vi "test-DiffOdometry.vi"() -> ()   [LabVIEW 2019]
uses:
  POSE.ctl
  TRANSLATION.ctl
  ROTATION.ctl
  PATH_SAMPLE.ctl
  PathExecution_Library.lvlib
panel:
  in  "Ramsete Enable":bool=TRUE
  in  "WheelBase-Feet":dbl
  in  "Path Sample":T1
  out "RightDmd FT/SEC":dbl
  out "LeftDMD Ft?SEC":dbl
  out "Heading DEG":dbl
  out "AtReference":bool
  out "Y Feet":dbl
  out "X Feet":dbl
  out "CurrentRelativePose":T2
  in  "Reset":bool
  in  "Gyro-Deg":dbl
  in  "RightDist-Feet":dbl
  in  "LeftDist-Feet":dbl
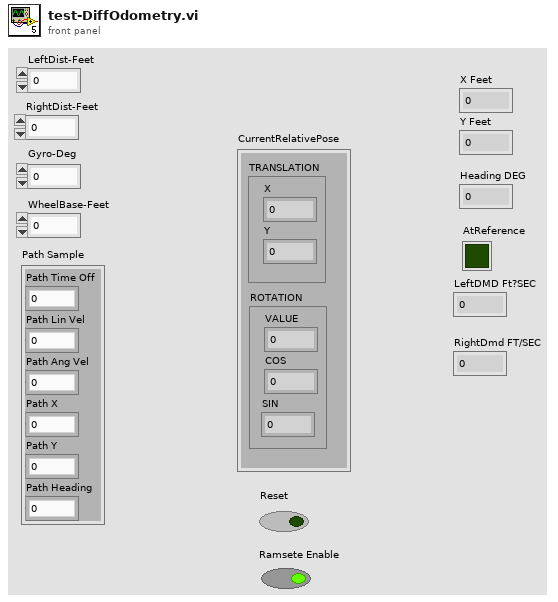
[diagram p1: front panel]
types:
  T1 = typedef "PathExecution_Library.lvlib/PATH_SAMPLE.ctl" = cluster{"Path Lin Vel":dbl, "Path Ang Vel":dbl, "Path X":dbl, "Path Y":dbl, "Path Heading":dbl, "Path Time Off":dbl}
  T2 = typedef "PathExecution_Library.lvlib/POSE.ctl" = cluster{"TRANSLATION":T3, "ROTATION":T4}
  T3 = typedef "PathExecution_Library.lvlib/TRANSLATION.ctl" = cluster{"X":dbl, "Y":dbl}
  T4 = typedef "PathExecution_Library.lvlib/ROTATION.ctl" = cluster{"VALUE":dbl, "COS":dbl, "SIN":dbl}
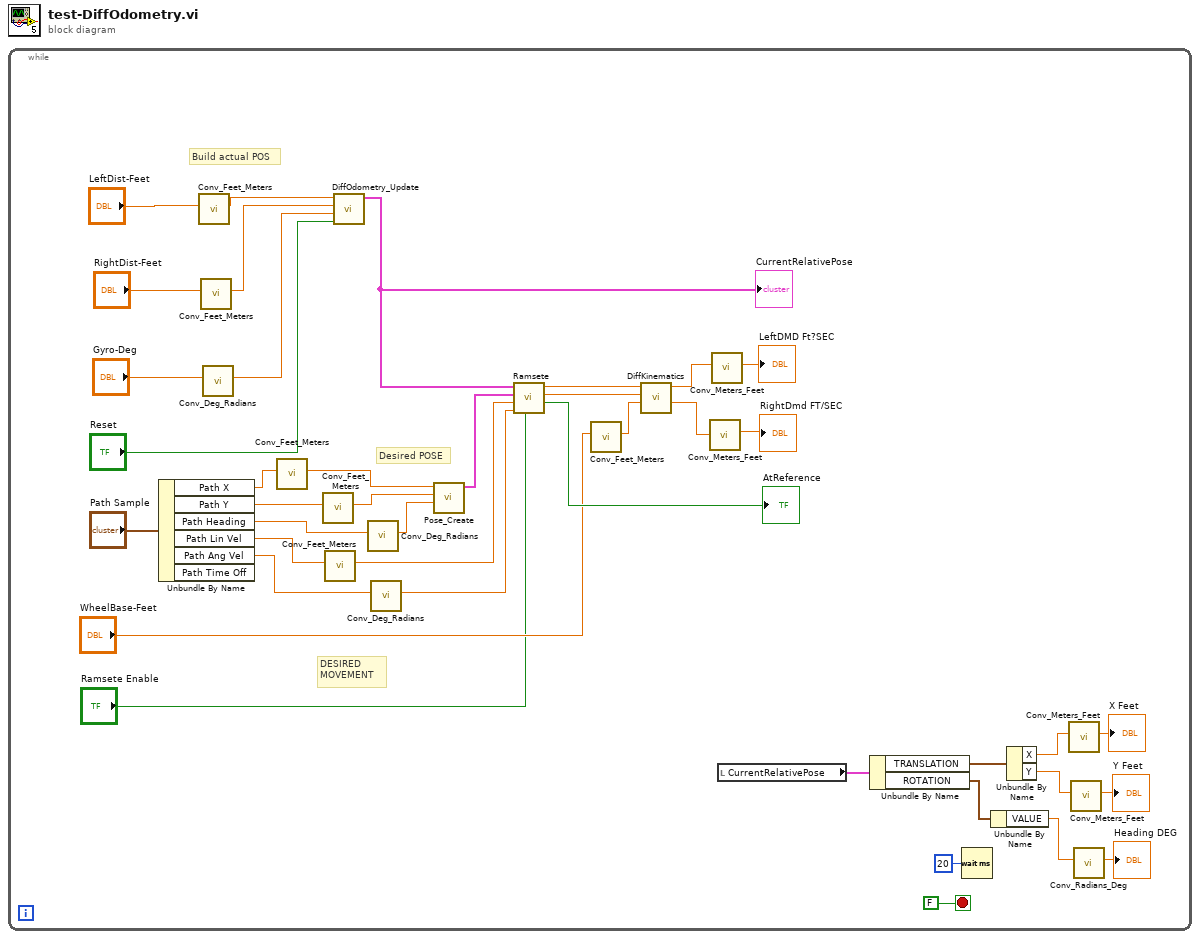
[diagram p0: block diagram]
diagram:
  n1 = while {
    stop <- FALSE stop-if-true
    # "DESIRED\nMOVEMENT"
    # "Desired POSE"
    # "Build actual POS"
    n2 = Unbundle By Name("Path Sample") -> ("Path X"=w11:dbl, "Path Y"=w9:dbl, "Path Heading"=w7:dbl, "Path Lin Vel"=w5:dbl, "Path Ang Vel"=w4:dbl)  [unwired: 1 out]
    n3 = call "Conv_Feet_Meters.vi"("Feet"="LeftDist-Feet") -> ("Meters"=w34:dbl)  [unwired: 10 in]
    n4 = call "Conv_Feet_Meters.vi"("Feet"="RightDist-Feet") -> ("Meters"=w28:dbl)  [unwired: 10 in]
    n5 = call "Conv_Deg_Radians.vi"("Degress"="Gyro-Deg") -> ("Radians"=w35:dbl)  [unwired: 10 in]
    n6 = call "Conv_Feet_Meters.vi"("Feet"=w11) -> ("Meters"=w10:dbl)  [unwired: 10 in]
    n7 = call "Conv_Feet_Meters.vi"("Feet"=w9) -> ("Meters"=w8:dbl)  [unwired: 10 in]
    n8 = call "Conv_Feet_Meters.vi"("Feet"=w5) -> ("Meters"=w3:dbl)  [unwired: 10 in]
    n9 = call "DiffOdometry_Update.vi"("Reset"="Reset", "GyroContinuous"=w35, "RightDistance"=w28, "LeftDistance"=w34) -> ("CurrentRelativePose"=w27:T2)  [unwired: 7 in]
    "CurrentRelativePose" <- w27
    n10 = call "Conv_Deg_Radians.vi"("Degress"=w7) -> ("Radians"=w6:dbl)  [unwired: 10 in]
    n11 = call "Conv_Deg_Radians.vi"("Degress"=w4) -> ("Radians"=w2:dbl)  [unwired: 10 in]
    n12 = call "Pose_Create.vi"("Heading"=w6, "Y"=w8, "X"=w10) -> ("out POSe"=w14:T2)  [unwired: 8 in]
    n13 = call "Ramsete.vi"("Enabled"="Ramsete Enable", "DesiredAngularVelocity"=w2, "DesiredLinearVelocity"=w3, "DesiredPOSE"=w14, "CurrentPOSE"=w27) -> ("AtReference"=→"AtReference":bool, "DemandAngularVelocity"=w21:dbl, "DemandLinearVelocity"=w22:dbl)  [unwired: 4 in]
    n14 = call "Conv_Feet_Meters.vi"("Feet"="WheelBase-Feet") -> ("Meters"=w20:dbl)  [unwired: 10 in]
    n15 = call "DiffKinematics.vi"("TrackWidth_Meters"=w20, "AngularVelocity"=w21, "LinearVelocity"=w22) -> ("RightVelocity"=w18:dbl, "LeftVelocity"=w19:dbl)  [unwired: 7 in]
    n16 = call "Conv_Meters_Feet.vi"("Meters"=w18) -> ("Feet"=→"RightDmd FT/SEC":dbl)  [unwired: 10 in]
    n17 = call "Conv_Meters_Feet.vi"("Meters"=w19) -> ("Feet"=→"LeftDMD Ft?SEC":dbl)  [unwired: 10 in]
    n18 = local read "CurrentRelativePose"() -> (w12:T2)
    n19 = Unbundle By Name(w12) -> ("TRANSLATION"=w33:T3, "ROTATION"=w25:T4)
    n20 = Wait (ms)(milliseconds to wait=u32 20) -> ()  [unwired: 1 out]
    n21 = Unbundle By Name(w25) -> ("VALUE"=w24:dbl)
    n22 = Unbundle By Name(w33) -> ("X"=w32:dbl, "Y"=w31:dbl)
    n23 = call "Conv_Meters_Feet.vi"("Meters"=w32) -> ("Feet"=→"X Feet":dbl)  [unwired: 10 in]
    n24 = call "Conv_Meters_Feet.vi"("Meters"=w31) -> ("Feet"=→"Y Feet":dbl)  [unwired: 10 in]
    n25 = call "Conv_Radians_Deg.vi"("Radians"=w24) -> ("Degrees"=→"Heading DEG":dbl)  [unwired: 10 in]
  }
